vi "AutoSet_Table_column1.vi"() -> ()   [LabVIEW 2021]
panel:
  in  "Table":string[][](table)=[["aaaaaaaaaaa", "wer we qewrwer ", "wer ", "qwe r", "qwe rweqrwer", "were", "qwe rweqr "], ["a", "werwe", "", "", "", "", ""], ["aaaaaaaaaaaaaaaa", "", "", "", "asdf asd", "asd fsdf a", "dfa sdfasdfsdf asdf"]]
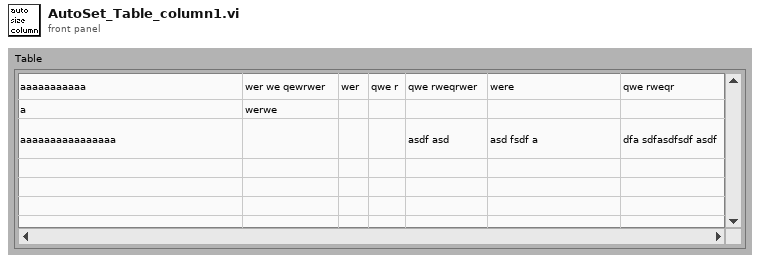
[diagram p1: front panel]
types:
  T1 = enum16{"User-specified Font", "Application Font", "System Font", "Dialog Font"}
  T2 = cluster{"Font Name:":string, "Size":i16, "Strikeout?":bool, "Italic?":bool, "Underline?":bool, "Outline?":bool, "Shadow?":bool, "Bold?":bool}
  T3 = cluster{"left":i16, "top":i16, "right":i16, "bottom":i16}
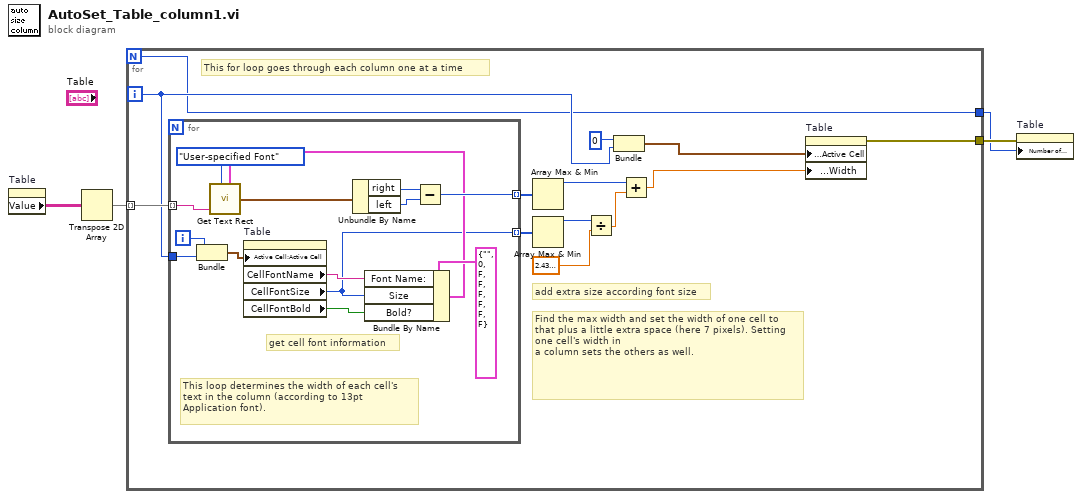
[diagram p0: block diagram]
diagram:
  n1 = property on="Table" class="Tbl (strict)"() -> ("Value"=w4:string[][])  [unwired: 2 in, 2 out]
  n2 = Transpose 2D Array(2D array=w4) -> (transposed array=w3:string[][])
  n3 = for {
    N -> [w5]
    tunnel: w3 -> [w17] mode=indexing
    tunnel: [w6] -> w2
    tunnel: [w5] -> w1
    i -> [w12]
    # "add extra size according font size"
    # "Find the max width and set the width of one cell to that plus a little extra space (here 7 pixels). Setting one cell's width in\na column sets the others as well."
    # "This for loop goes through each column one at a time"
    n4 = for {
      tunnel: w17 -> [w31] mode=indexing
      tunnel: [w27] -> w16 mode=indexing
      tunnel: w12 -> [w21]
      tunnel: [w18] -> w10 mode=indexing
      i -> [w20]
      # "get cell font information"
      # "This loop determines the width of each cell's\ntext in the column (according to 13pt\nApplication font)."
      n5 = Bundle(w20, w21) -> (w26:cluster{i32, i32})  [unwired: 1 in]
      n6 = property on="Table" class="Tbl (strict)"("Active Cell:Active Cell"=w26) -> ("CellFontName"=w25:string, "CellFontSize"=w18:u32, "CellFontBold"=w24:bool)  [unwired: 2 in, 2 out]
      n7 = Bundle By Name(cluster=T2 {"Font Name:"="", "Size"=0, "Strikeout?"=FALSE, "Italic?"=FALSE, "Underline?"=FALSE, "Outline?"=FALSE, "Shadow?"=FALSE, "Bold?"=FALSE} ("[user-specified font]"), "Font Name:"=w25, "Size"=w18, "Bold?"=w24) -> (w22:T2)
      n8 = call <vilib>:"Get Text Rect.vi"("desired font(Application)"=T1."User-specified Font", "text"=w31, "[user-specified font]"=w22) -> ("rect"=w30:T3)  [unwired: 6 in]
      n9 = Unbundle By Name(w30) -> ("right"=w29:i16, "left"=w28:i16)
      n10 = Subtract(x=w29, y=w28) -> (x-y=w27:i16)
    }
    n11 = Array Max & Min(array=w16) -> (max value=w11:i16)  [unwired: 3 out]
    n12 = Array Max & Min(array=w10) -> (max value=w9:u32)  [unwired: 3 out]
    n13 = Divide(x=w9, y=sgl 2.43) -> (x/y=w7:sgl)
    n14 = Bundle(0, w12) -> (w13:cluster{i32, i32})  [unwired: 1 in]
    n15 = Add(x=w11, y=w7) -> (x+y=w14:sgl)
    n16 = property on="Table" class="Tbl (strict)"("Active Cell:Active Cell"=w13, "Active Cell:Cell Size:Width"=w14) -> (error out=w6:errorcluster)  [unwired: 2 in, 1 out]
  }
  n17 = property on="Table" class="Tbl (strict)"(error in=w2, "Number of Columns"=w1) -> ()  [unwired: 1 in, 2 out]
